vi "Read from Dashboard.vi"() -> ()   [LabVIEW 2017]
uses:
  <vilib>/Rock Robotics/Network Tables/NT Read Number.vi
panel:
  in  "Teleop Controls":T1(tab)
  in  "Y Axis":T2
  in  "X Axis":T2
  in  "Forward Trim":T3={"Trim Max"=0.37, "Trim Min"=0.01, "Trim Deadzone"=0.1, "Trim LR"=TRUE}
  in  "Backward Trim":T3={"Trim Max"=0.5, "Trim Min"=0.05, "Trim Deadzone"=0.1, "Trim LR"=FALSE}
  in  "PID Tuning":enum32{"Drive with PID", "Turn by Angle"}(tab)
  in  "Drive with PID":T4={"Max Speed"=0.7, "P/I/D"=[1.0, 0.0, 0.01], "Min Speed"=0.4, "Accel Distance"=64.0}
  in  "Turn By Angle":T5={"P/I/D"=[0.25, 0.001, 0.0], "Turn Speed"=0.55, "Linearity"=0.6}
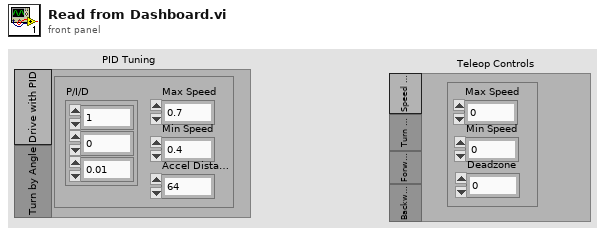
[diagram p1: front panel]
types:
  T1 = enum32{"Speed Sensitivity", "Turn Sensitivity", "Forward Trim", "Backwards Trim"}
  T2 = cluster{"Max Speed":dbl, "Min Speed":dbl, "Deadzone":dbl}
  T3 = cluster{"Trim Max":dbl, "Trim Min":dbl, "Trim Deadzone":dbl, "Trim LR":bool}
  T4 = cluster{"Max Speed":dbl, "P/I/D":dbl[], "Min Speed":dbl, "Accel Distance":dbl}
  T5 = cluster{"P/I/D":dbl[], "Turn Speed":dbl, "Linearity":dbl}
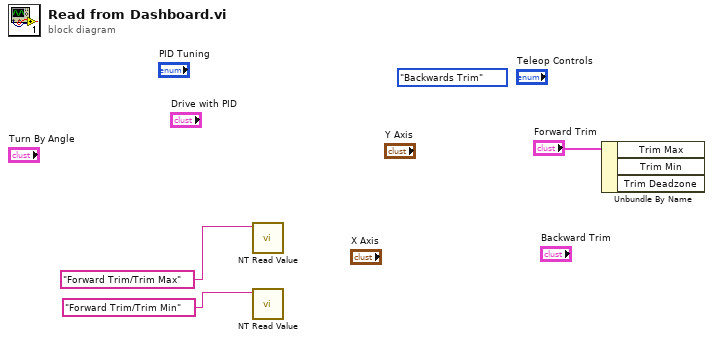
[diagram p0: block diagram]
diagram:
  (unwired) T1."Backwards Trim" ("Teleop Controls")
  n1 = call-poly <vilib>:"NT Read Value.vi"("Name"="Forward Trim/Trim Max") -> ("Numeric"=w3:dbl)  [unwired: 9 in, 1 out]
  n2 = call-poly <vilib>:"NT Read Value.vi"("Name"="Forward Trim/Trim Min") -> ("Numeric"=w4:dbl)  [unwired: 9 in, 1 out]
  n3 = Unbundle By Name("Forward Trim") -> ()  [unwired: 3 out]
